vi "convert_boolean_to_ON_OFF_string.vi"(4 "boolean value in":bool, 5 "String to add before (\"\")":string) -> (1 "string value out":string)   [LabVIEW 2020, in "Rohde&Schwarz RTx Oscilloscopes.lvlib" / "rsidr_core.lvlib"]
uses:
  rsidr_core.lvlib
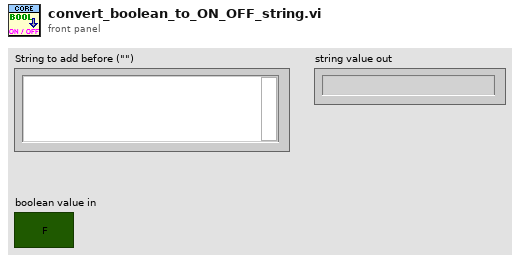
[diagram p1: front panel]
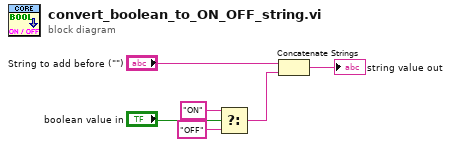
[diagram p0: block diagram]
diagram:
  n1 = Select(t="ON" ("search string/char (-)"), s="boolean value in", f="OFF" ("search string/char (-)")) -> (s? t:f=w2:string)
  n2 = Concatenate Strings("String to add before (\"\")", w2) -> (→"string value out":string)
